vi "App Config INI.vi"(8 "error in (no error)":errorcluster) -> (0 "error out":errorcluster, 3 "App Config":path)   [LabVIEW 2020, in "MacroAssert.lvlib"]
uses:
  MacroAssert.lvlib
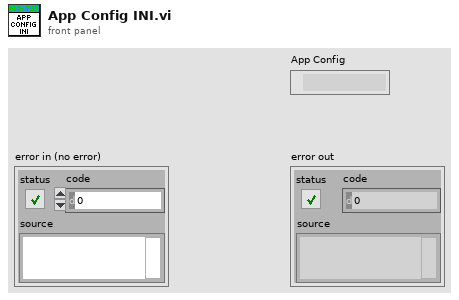
[diagram p1: front panel]
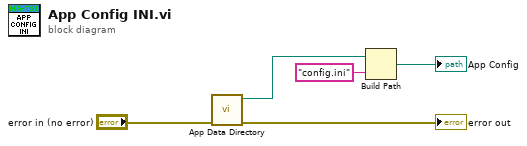
[diagram p0: block diagram]
diagram:
  n1 = call "App Data Directory.vi"("error in (no error)"="error in (no error)") -> ("error out"=→"error out":errorcluster, "App Data Directory"=w3:path)  [unwired: 9 in]
  n2 = Build Path(base path=w3, name or relative path="config.ini") -> (appended path=→"App Config":path)
